vi "UpdateWeightsHidden2.vi"(0 "OutH1":sgl[](array[numeric]), 5 "OutH2":sgl[](array[numeric])=[0.0, 0.0, 0.0, 0.0], 7 "Output":sgl, 9 "dEtot_dOut":sgl, 11 "Learning Rate":sgl) -> ()   [LabVIEW 2020]
uses:
  <vilib>/rvi/Emulation/niFpgaSctlEmulationGetInTimedLoop.vi
  Global var FPGA.vi
  <vilib>/rvi/Memory/Memory_Emulation/nirvimemoryFastEmulation.vi
  <vilib>/rvi/Memory/Memory_Emulation/nirvimemoryEmulation.vi
  <vilib>/rvi/Emulation/niFpgaEmulationIsFPGAContextNoSignature.vi
  <vilib>/rvi/DataTransferAndStorage/Container/Common/niFpgaContainerGetUniqueNameForEmu.vi
  <vilib>/rvi/Emulation/niFpgaProcessEmulError.vi
  <vilib>/rvi/errors/nirviReportUnexpectedCaseInternalError (U32).vi
  <vilib>/rvi/DataTransferAndStorage/Container/XNode/niFpgaContainer.xnode
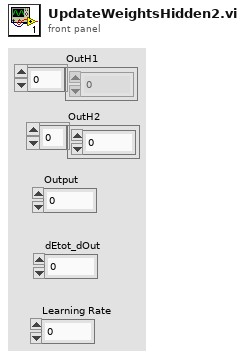
[diagram p1: front panel]
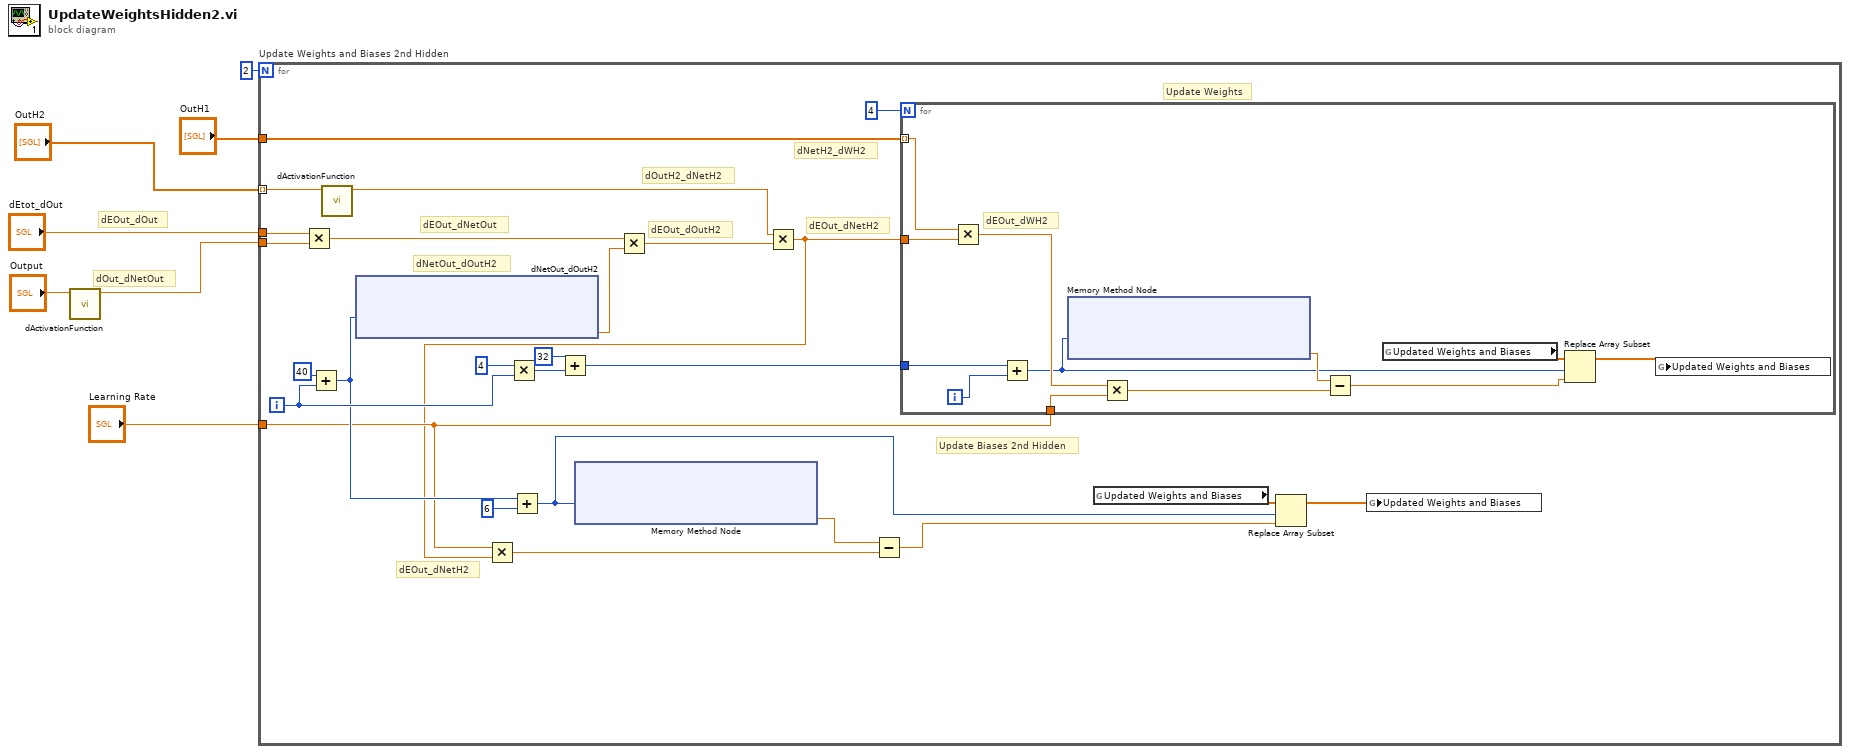
[diagram p0: block diagram]
diagram:
  # "dEOut_dOut"
  # "dOut_dNetOut"
  n1 = call "dActivationFunction.vi"("Output"="Output") -> ("f"=w3:sgl)  [unwired: 10 in]
  n2 = for "Update Weights and Biases 2nd Hidden" {
    N: 2 -> [_]
    tunnel: "OutH2" -> [w17] mode=indexing
    tunnel: w3 -> [w32]
    tunnel: "dEtot_dOut" -> [w31]
    tunnel: "Learning Rate" -> [w20]
    tunnel: "OutH1" -> [w18]
    i -> [w25]
    # "Update Weights"
    # "dEOut_dNetH2"
    # "dEOut_dNetH2"
    # "dEOut_dOutH2"
    # "dNetH2_dWH2"
    # "dOutH2_dNetH2"
    # "dNetOut_dOutH2"
    # "dEOut_dNetOut"
    # "Update Biases 2nd Hidden"
    n3 = Multiply(x=w31, y=w32) -> (x*y=w15:sgl)
    n4 = Add(x=40, y=w25) -> (x+y=w23:i32)
    n5 = call "dActivationFunction.vi"("Output"=w17) -> ("f"=w13:sgl)  [unwired: 10 in]
    n6 = xnode ("dNetOut_dOutH2")("Address"=w23) -> ("Data"=w16:sgl)  [unwired: 1 in, 1 out]
    n7 = Multiply(x=4, y=w25) -> (x*y=w27:i32)
    n8 = Add(x=w23, y=6) -> (x+y=w9:i32)
    n9 = Add(x=u32 32 ("Address"), y=w27) -> (x+y=w28:u32)
    n10 = xnode ("Memory Method Node")("Address"=w9) -> ("Data"=w19:sgl)  [unwired: 1 in, 1 out]
    n11 = Multiply(x=w15, y=w16) -> (x*y=w14:sgl)
    n12 = Multiply(x=w13, y=w14) -> (x*y=w12:sgl)
    n13 = Multiply(x=w20, y=w12) -> (x*y=w21:sgl)
    n14 = Subtract(x=w19, y=w21) -> (x-y=w8:sgl)
    n15 = for {
      N: 4 -> [_]
      tunnel: w28 -> [w44]
      tunnel: w20 -> [w42]
      tunnel: w18 -> [w37] mode=indexing
      tunnel: w12 -> [w38]
      i -> [w43]
      # "dEOut_dWH2"
      n16 = Multiply(x=w37, y=w38) -> (x*y=w41:sgl)
      n17 = Add(x=w44, y=w43) -> (x+y=w34:u32)
      n18 = xnode ("Memory Method Node")("Address"=w34) -> ("Data"=w40:sgl)  [unwired: 1 in, 1 out]
      n19 = Multiply(x=w41, y=w42) -> (x*y=w39:sgl)
      n20 = Subtract(x=w40, y=w39) -> (x-y=w33:sgl)
      n21 = global read "Global var FPGA.vi" "Updated Weights and Biases"() -> (w36:sgl[])
      n22 = Replace Array Subset(array=w36, new element=w33, index=w34) -> (w35:sgl[])
      n23 = global write "Global var FPGA.vi" "Updated Weights and Biases"(w35) -> ()
    }
    n24 = global read "Global var FPGA.vi" "Updated Weights and Biases"() -> (w11:sgl[])
    n25 = Replace Array Subset(array=w11, new element=w8, index=w9) -> (w10:sgl[])
    n26 = global write "Global var FPGA.vi" "Updated Weights and Biases"(w10) -> ()
  }
